vi "HAL camera program for acquisition.vi"(2 "error in":errorcluster, 3 "Camera Parameters (important)":T1={"Exposure Time (sec)"=0.0, "Readout Settings"={"Per-pixel gain compensation"=TRUE, "Readout speed"=TRUE}, "Image Size"={"Left"=0, "Top"=0, "Right"=1, "Bottom"=0, "Binning"=1}} {"Image Size"."Binning" items=["1 x 1"=1, "2 x 2"=2, "4 x 4"=4]; "Image Size"."Bottom" min=4 max=2048 step=4; "Image Size"."Right" min=4 max=2048 step=4; "Image Size"."Top" min=1 max=2048 step=4; "Image Size"."Left" min=1 max=2048 step=4; "Exposure Time (sec)" scale=0.001..10.0 scale format="%#_1g"}) -> (0 "error out":errorcluster, 1 "Actual Exposure Time (sec)":sgl)   [LabVIEW 2011]
uses:
  HAL camera parameters important.ctt
  orca readout settings.ctl
  image size.ctl
  HAL Camera specifications globals.vi
  Camera/camera globals.vi
panel:
  out "Image Size.Binning":u16
  # "Camera: Hammamatsu Orca"
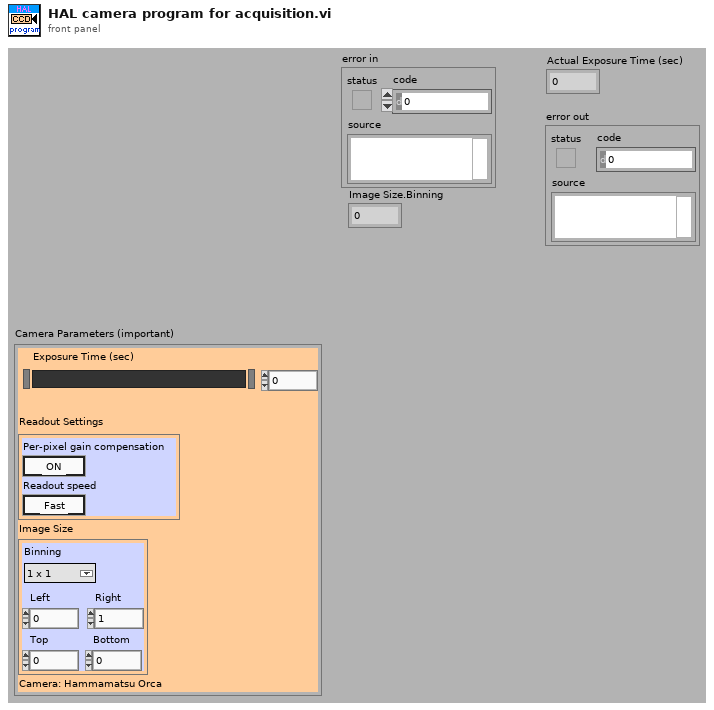
[diagram p1: front panel]
types:
  T1 = typedef "HAL camera parameters important.ctt" = cluster{"Exposure Time (sec)":sgl, "Readout Settings":T2, "Image Size":T3}
  T2 = typedef "orca readout settings.ctl" = cluster{"Per-pixel gain compensation":bool, "Readout speed":bool}
  T3 = typedef "image size.ctl" = cluster{"Left":i32, "Top":i32, "Right":i32, "Bottom":i32, "Binning":u16}
  T4 = cluster{"Horizontal Offset":i32, "Vertical Offset":i32, "Horizontal Width":i32, "Vertical Width":i32}
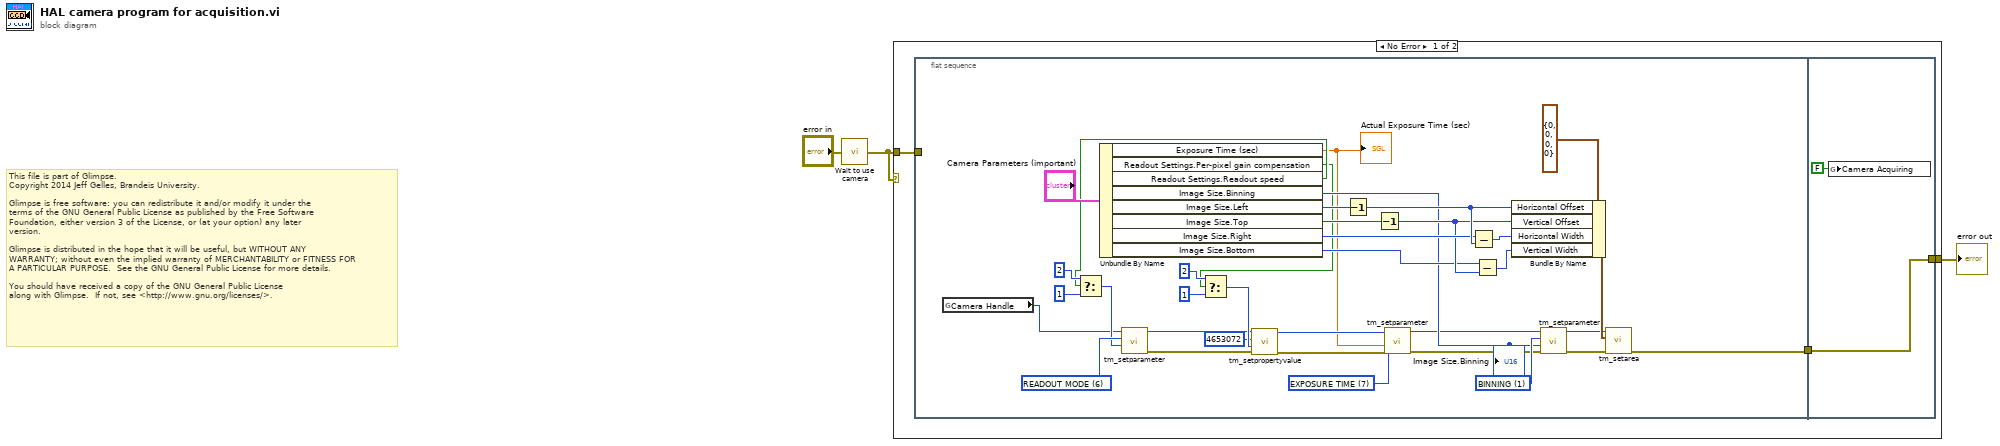
[diagram p0: block diagram]
diagram:
  # "This file is part of Glimpse. \nCopyright 2014 Jeff Gelles, Brandeis University.    \n\nGlimpse is free software: you can redistribute it and/or modify it under the \nterms of the GNU General Public License as published by the Free Software \nFoundation, either version 3 of the License, or (at your option) any later \nversion.\n\nGlimpse is distributed in the hope that it will be useful, but WITHOUT ANY \nWARRANTY; without even the implied warranty of MERCHANTABILITY or FITNESS FOR \nA PARTICULAR PURPOSE.  See the GNU General Public License for more details.\n\nYou should have received a copy of the GNU General Public License\nalong with Glimpse.  If not, see <http://www.gnu.org/licenses/>."
  n1 = call "Wait to use camera.vi"("error in"="error in") -> ("error out"=w1:errorcluster)
  n2 = case shown="No Error" w1 {
    tunnel: [w5 w44] -> w3
    tunnel: w1 -> [w6 w44]
    frame No Error {
      n3 = flat-sequence {
        tunnel: w6 -> [_]
        tunnel: [w7] -> w4
        tunnel: [w42] -> w5
        tunnel: w4 -> [w42]
        frame #0 {
          w19 = 7 items=["BINNING"=1, "BITS PER CHANNEL"=2, "ACTIVE VIEW INDEX"=3, "CCD MODE"=4, "SENSOR MODE"=5, "READOUT MODE"=6, "EXPOSURE TIME"=7, "CONTRAST GAIN"=8, "CONTRAST OFFSET"=9, "LIGHT MODE"=10, "SENSITIVITY"=11, "WHITE BALANCE"=12, "PHOTON IMAGING MODE"=13, "HIGH DYNAMIC RANGE MODE"=14, "TRIGGER SOURCE"=15, "TRIGGER ACTIVE"=16, "TRIGGER MODE"=17, "TRIGGER POLARITY"=18, "TRIGGER GLOBAL EXPOSURE"=19, "FIRST TRIGGER BEHAVIOR"=20, "TRIGGER TIMES"=21, "OUTPUT TRIGGER POLARITY"=22, "OUTPUT TRIGGER DELAY"=23, "OUTPUT TRIGGER PERIOD"=24, "TEMPERATURE"=25, "TEMPERATURE TARGET"=26, "SENSOR COOLER FAN"=27, "MECHANICAL SHUTTER"=28, "BACK FOCUS POSITION"=29, "FRAMEBUNDLE MODE"=30, "FRAMEBUNDLE NUMBER"=31, "LINEBUNDLE HEIGHT"=32, "TRIGGER CONNECTOR"=33, "IMAGE PIXEL TYPE"=34] ("Parameter")
          w28 = 6 items=["BINNING"=1, "BITS PER CHANNEL"=2, "ACTIVE VIEW INDEX"=3, "CCD MODE"=4, "SENSOR MODE"=5, "READOUT MODE"=6, "EXPOSURE TIME"=7, "CONTRAST GAIN"=8, "CONTRAST OFFSET"=9, "LIGHT MODE"=10, "SENSITIVITY"=11, "WHITE BALANCE"=12, "PHOTON IMAGING MODE"=13, "HIGH DYNAMIC RANGE MODE"=14, "TRIGGER SOURCE"=15, "TRIGGER ACTIVE"=16, "TRIGGER MODE"=17, "TRIGGER POLARITY"=18, "TRIGGER GLOBAL EXPOSURE"=19, "FIRST TRIGGER BEHAVIOR"=20, "TRIGGER TIMES"=21, "OUTPUT TRIGGER POLARITY"=22, "OUTPUT TRIGGER DELAY"=23, "OUTPUT TRIGGER PERIOD"=24, "TEMPERATURE"=25, "TEMPERATURE TARGET"=26, "SENSOR COOLER FAN"=27, "MECHANICAL SHUTTER"=28, "BACK FOCUS POSITION"=29, "FRAMEBUNDLE MODE"=30, "FRAMEBUNDLE NUMBER"=31, "LINEBUNDLE HEIGHT"=32, "TRIGGER CONNECTOR"=33, "IMAGE PIXEL TYPE"=34] ("Parameter")
          w30 = 1 items=["BINNING"=1, "BITS PER CHANNEL"=2, "ACTIVE VIEW INDEX"=3, "CCD MODE"=4, "SENSOR MODE"=5, "READOUT MODE"=6, "EXPOSURE TIME"=7, "CONTRAST GAIN"=8, "CONTRAST OFFSET"=9, "LIGHT MODE"=10, "SENSITIVITY"=11, "WHITE BALANCE"=12, "PHOTON IMAGING MODE"=13, "HIGH DYNAMIC RANGE MODE"=14, "TRIGGER SOURCE"=15, "TRIGGER ACTIVE"=16, "TRIGGER MODE"=17, "TRIGGER POLARITY"=18, "TRIGGER GLOBAL EXPOSURE"=19, "FIRST TRIGGER BEHAVIOR"=20, "TRIGGER TIMES"=21, "OUTPUT TRIGGER POLARITY"=22, "OUTPUT TRIGGER DELAY"=23, "OUTPUT TRIGGER PERIOD"=24, "TEMPERATURE"=25, "TEMPERATURE TARGET"=26, "SENSOR COOLER FAN"=27, "MECHANICAL SHUTTER"=28, "BACK FOCUS POSITION"=29, "FRAMEBUNDLE MODE"=30, "FRAMEBUNDLE NUMBER"=31, "LINEBUNDLE HEIGHT"=32, "TRIGGER CONNECTOR"=33, "IMAGE PIXEL TYPE"=34] ("Parameter")
          n4 = global read "HAL Camera specifications globals.vi" "Camera Handle"() -> (w9:u32)
          n5 = Unbundle By Name("Camera Parameters (important)") -> ("Exposure Time (sec)"=w10:sgl, "Readout Settings.Per-pixel gain compensation"=w20:bool, "Readout Settings.Readout speed"=w24:bool, "Image Size.Binning"=w29:u16, "Image Size.Left"=w38:i32, "Image Size.Top"=w37:i32, "Image Size.Right"=w33:i32, "Image Size.Bottom"=w31:i32)
          "Actual Exposure Time (sec)" <- w10
          "Image Size.Binning" <- w29
          n6 = Select(t=i16 2 ("f"), s=w24, f=i16 1) -> (s? t:f=w27:i16)
          n7 = call <userlib>:"tm_setparameter.vi"("Value in"=w27, "Parameter"=w28, "Handle in"=w9) -> ("error out"=w18:errorcluster, "Handle out"=w14:u32)  [unwired: 7 in]
          n8 = Select(t=i16 2 ("f"), s=w20, f=i16 1) -> (s? t:f=w21:i16)
          n9 = call <userlib>:"tm_setpropertyvalue.vi"("error in (no error)"=w18, "Value in"=w21, "Property ID"=u32 4653072, "Handle in"=w14) -> ("error out"=w17:errorcluster, "Handle out"=w13:u32)  [unwired: 6 in]
          n10 = Decrement(x=w38) -> (x-1=w34:i32)
          n11 = Decrement(x=w37) -> (x-1=w32:i32)
          n12 = call <userlib>:"tm_setparameter.vi"("error in (no error)"=w17, "Value in"=w10, "Parameter"=w19, "Handle in"=w13) -> ("error out"=w16:errorcluster, "Handle out"=w12:u32)  [unwired: 6 in]
          n13 = Subtract(x=w33, y=w34) -> (x-y=w36:i32)
          n14 = Subtract(x=w31, y=w32) -> (x-y=w35:i32)
          n15 = Bundle By Name(cluster=T4 {"Horizontal Offset"=0, "Vertical Offset"=0, "Horizontal Width"=0, "Vertical Width"=0} ("Sub Region"), "Horizontal Offset"=w34, "Vertical Offset"=w32, "Horizontal Width"=w36, "Vertical Width"=w35) -> (w40:T4)
          n16 = call <userlib>:"tm_setparameter.vi"("error in (no error)"=w16, "Value in"=w29, "Parameter"=w30, "Handle in"=w12) -> ("error out"=w15:errorcluster, "Handle out"=w11:u32)  [unwired: 6 in]
          n17 = call <userlib>:"tm_setarea.vi"("error in (no error)"=w15, "Sub Region"=w40, "Handle in"=w11) -> ("error out"=w7:errorcluster)  [unwired: 7 in, 1 out]
        }
        frame #1 {
          n18 = global write "camera globals.vi" "Camera Acquiring"(FALSE ("Andor Aquiring")) -> ()
        }
      }
    }
    frame Error {
    }
  }
  "error out" <- w3
